vi "Rename Event.vi"(8 "error in (no error)":errorcluster, 9 "New Name":string, 10 "Old Name":string, 11 "State in":refnum<class "State.lvclass">) -> (0 "error out":errorcluster, 3 "State out":refnum<class "State.lvclass">)   [LabVIEW 2015, in "State.lvclass"]
uses:
  State.lvclass
  State.lvclass/State.ctl
  Termination/Termination.lvclass
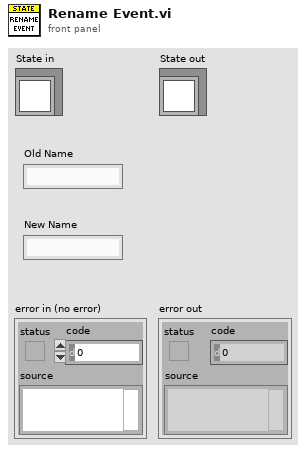
[diagram p1: front panel]
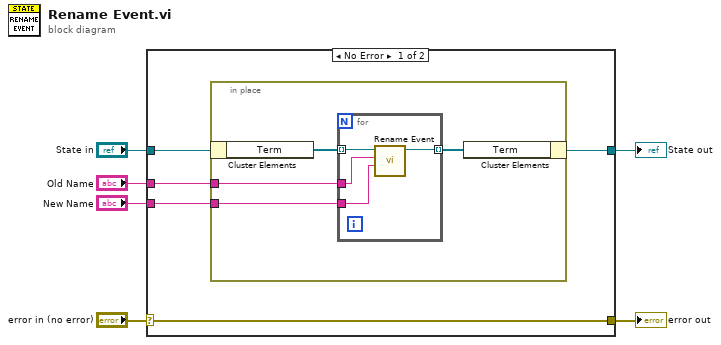
[diagram p0: block diagram]
diagram:
  n1 = case shown="No Error" "error in (no error)" {
    selector: "error in (no error)" -> [w11 w21]
    tunnel: [w11 w21] -> w5
    tunnel: [w9 w20] -> w3
    tunnel: "State in" -> [w10 w20]
    tunnel: "Old Name" -> [w8 _]
    tunnel: "New Name" -> [w7 _]
    frame No Error {
      n2 = in-place {
        in-place-border: w8 -> [w13]
        in-place-border: w7 -> [w12]
        n3 = in-place-cluster #1(w10) -> ("Term"=w15:refnum<class "Termination.lvclass">[])
        n4 = for {
          tunnel: w15 -> [w19] mode=indexing
          tunnel: [w16] -> w14 mode=indexing
          tunnel: w13 -> [w18]
          tunnel: w12 -> [w17]
          n5 = call "Rename Event.vi"("New Name"=w17, "Old Name"=w18, "Termination in"=w19) -> ("Termination out"=w16:refnum<class "Termination.lvclass">)  [unwired: 7 in, 1 out]
        }
        n6 = in-place-cluster #1("Term"=w14) -> (w9:refnum<class "State.lvclass">)
      }
    }
    frame Error {
    }
  }
  "error out" <- w5
  "State out" <- w3
